vi "test Array from Owned Array.vi"(8 "error in (no error)":errorcluster, 11 "TestCase in":refnum<class "Data Structure Tests.lvclass">) -> (0 "error out":errorcluster, 3 "TestCase out":refnum<class "Data Structure Tests.lvclass">)   [LabVIEW 2020, in "Data Structure Tests.lvclass"]
uses:
  Data Structure Tests.lvclass
  <vilib>/Utility/file.llb/Application Directory.vi
  <vilib>/Utility/libraryn.llb/Check if File or Folder Exists.vi
  <vilib>/addons/_JKI Toolkits/VI Tester/TestCase.llb/TestCase.lvclass
  C:/Program Files/National Instruments/LabVIEW 2024/vi.lib/addons/_JKI Toolkits/VI Tester/TestCase.llb/TestCase.lvclass
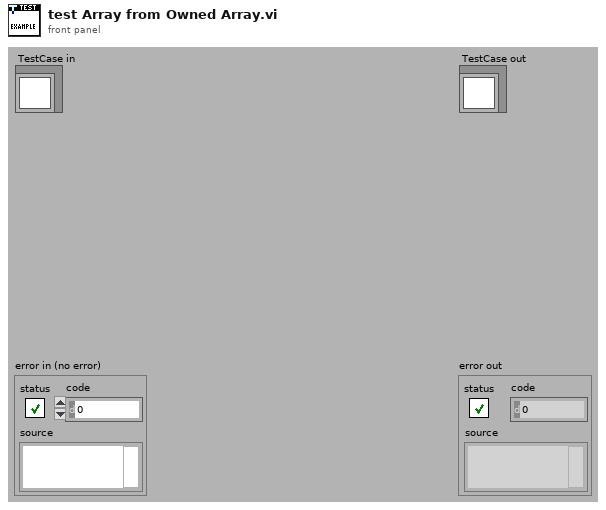
[diagram p1: front panel]
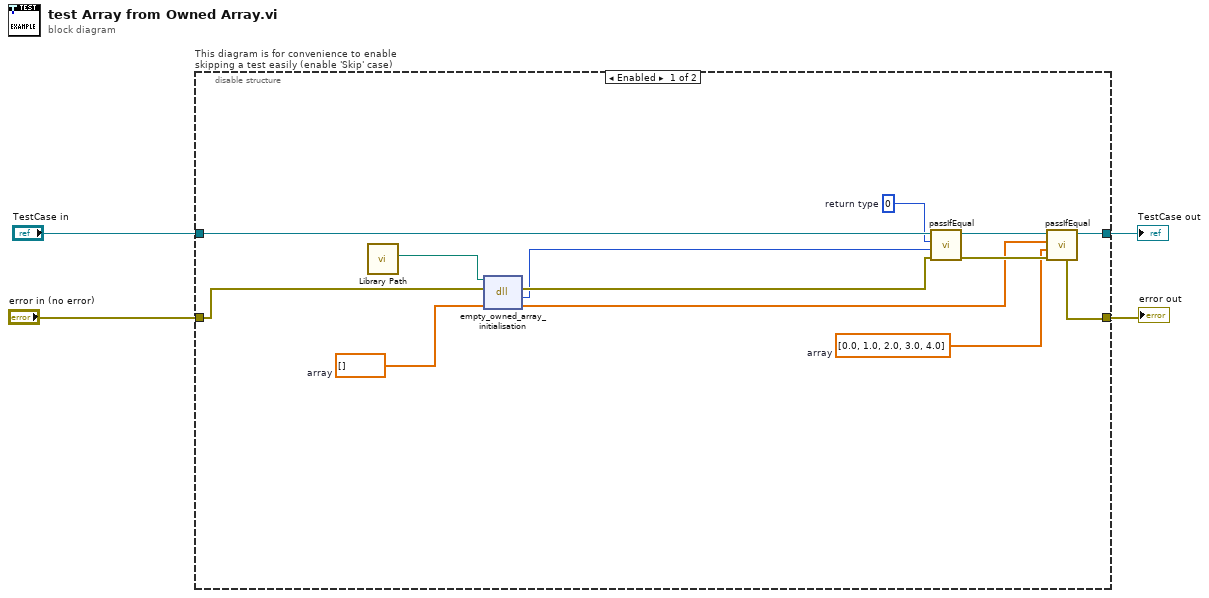
[diagram p0: block diagram]
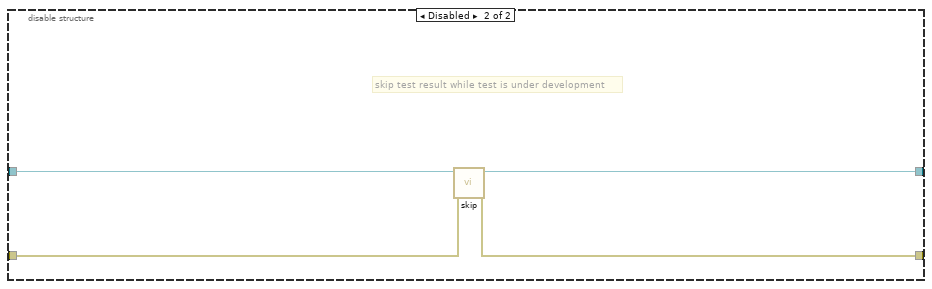
[diagram p2: hidden frame]
diagram:
  n1 = disable-structure "This diagram is for convenience to enable skipping a test easily (enable 'Skip' case)" shown="Enabled" {
    disable-tunnel: "TestCase in" -> [w17 w21]
    disable-tunnel: [w11 w19] -> w1
    disable-tunnel: [w13 w20] -> w3
    disable-tunnel: "error in (no error)" -> [w16 w18]
    frame Enabled {
      w5 = dbl[] [0.0, 1.0, 2.0, 3.0, 4.0]  # array
      w7 = 0  # return type
      w9 = dbl[] []  # array
      n2 = call "Library Path.vi"() -> ("Library Path"=w10:path)  [unwired: 11 in]
      n3 = dll-call lib="C:/Users/JamesMcNally/Documents/RustInterop/Rust-LabVIEW-Interop/target/debug/labview_test_library.dll" fn="empty_owned_array_initialisation"(path in=w10, error in=w16, "array"=w9) -> (error out=w15:errorcluster, "return type"=w8:i32, "array"=w6:dbl[])  [unwired: 1 in, 1 out]
      n4 = call-dynamic "passIfEqual.vi"("error in (no error)"=w15, "y"=w8, "x"=w7, "TestCase in"=w17) -> ("error out"=w14:errorcluster, "TestCase out"=w12:refnum<class "Data Structure Tests.lvclass">)  [unwired: 6 in]
      n5 = call-dynamic "passIfEqual.vi"("error in (no error)"=w14, "y"=w5, "x"=w6, "TestCase in"=w12) -> ("error out"=w13:errorcluster, "TestCase out"=w11:refnum<class "Data Structure Tests.lvclass">)  [unwired: 6 in]
    }
    frame Disabled {
      # "skip test result while test is under development"
      n6 = call <vilib>:"skip.vi"("error in (no error)"=w18, "TestCase in"=w21) -> ("error out"=w20:errorcluster, "TestCase out"=w19:refnum<class "Data Structure Tests.lvclass">)  [unwired: 8 in]
    }
  }
  "error out" <- w3
  "TestCase out" <- w1
